vi "CreateFormatter.vi"(4 "Validate":bool=TRUE, 5 "DateFormat":string, 6 "Style":string, 7 "Format":string, 8 "error in (no error)":errorcluster, 10 "Name":string, 11 "Logger in":refnum<class "Logger.lvclass">) -> (0 "error out":errorcluster, 2 "Formatter":refnum<class "Formatter.lvclass">, 3 "Logger out":refnum<class "Logger.lvclass">)   [LabVIEW 2022 SP3, in "Logger.lvlib" / "Logger.lvclass"]
uses:
  Logger.lvclass
  C:/Users/jakub/repos/gh/sw4sys/lv-logger/PythonWrapper/Source/PythonSession/PythonSession.lvclass
  C:/Users/jakub/repos/gh/sw4sys/lv-logger/PythonWrapper/Source/PythonWrapper/PythonWrapper.lvclass
  C:/Users/jakub/repos/gh/sw4sys/lv-logger/Logger/Source/LoggingWrapper/LoggingWrapper.lvclass
  Formatter/Formatter.lvclass
  PythonWrapper/Source/PythonSession/PythonSession.lvclass/PythonSession.ctl
  PythonWrapper/Source/PythonWrapper/PythonWrapper.lvclass/PythonWrapper.ctl
  LoggingWrapper/LoggingWrapper.lvclass/LoggingWrapper.ctl
  Formatter/Formatter.lvclass/Formatter.ctl
  Formatter/Write Name.vi
  PythonWrapper/Source/PythonSession/Read PythonSession.vi
  PythonWrapper/Source/PythonWrapper/Read ModulePath.vi
  PythonWrapper/Source/PythonSession/SessionBank.vi
  Logger.lvclass/Logger.ctl
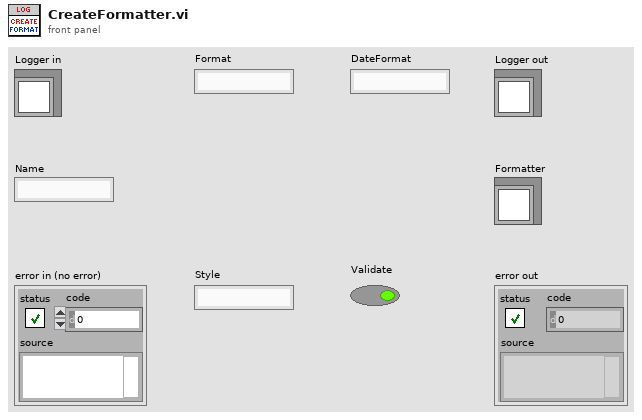
[diagram p1: front panel]
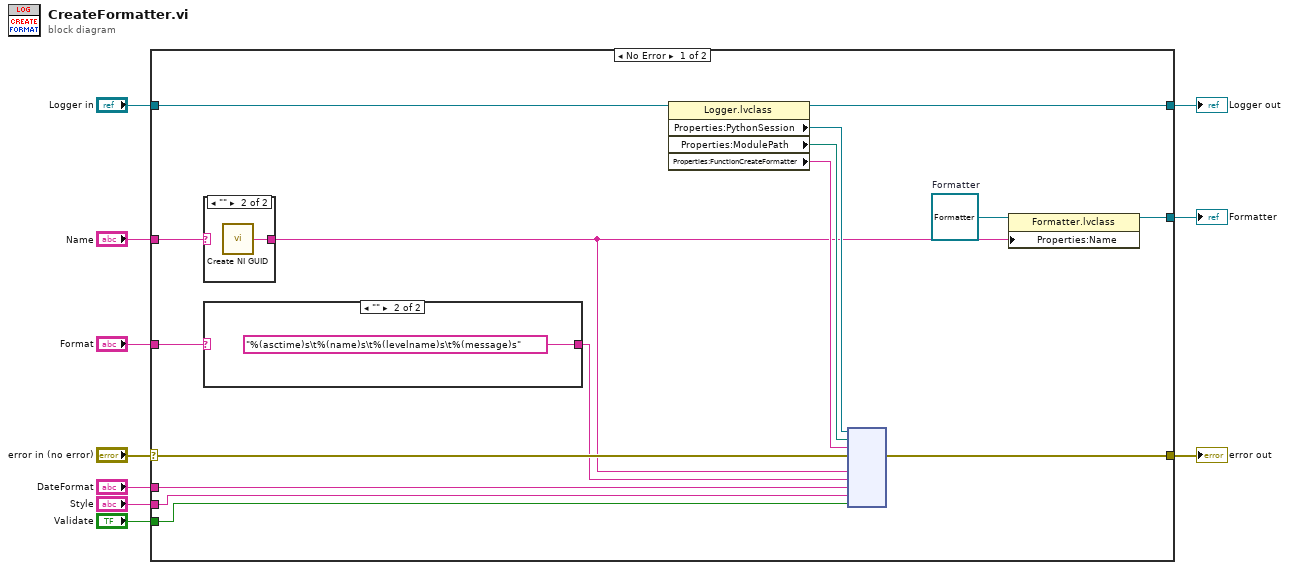
[diagram p0: block diagram]
diagram:
  n1 = case shown="No Error" "error in (no error)" {
    selector: "error in (no error)" -> [w20 w32]
    tunnel: [w19 w32] -> w6
    tunnel: [w17 w31] -> w8
    tunnel: "Logger in" -> [w22 w31]
    tunnel: "Format" -> [w21 _]
    tunnel: "DateFormat" -> [w13 _]
    tunnel: "Style" -> [w14 _]
    tunnel: "Validate" -> [w15 _]
    tunnel: [w16 _] -> w7
    tunnel: "Name" -> [w18 _]
    frame No Error {
      w23 = refnum<class "Formatter.lvclass"> refnum  # Formatter
      n2 = case shown="\"\"" w18 {
        selector: w18 -> [w29 _]
        tunnel: [w29 w30] -> w11
        frame Default {
        }
        frame "" {
          n3 = call <vilib>:"Create NI GUID.vi"() -> ("NI GUID"=w30:string)
        }
      }
      n4 = case shown="\"\"" w21 {
        selector: w21 -> [w27 _]
        tunnel: [w27 "%(asctime)s\t%(name)s\t%(levelname)s\t%(message)s"] -> w12
        frame Default {
        }
        frame "" {
        }
      }
      n5 = property class="Logger.lvclass"(reference=w22) -> (reference out=w17:refnum<class "Logger.lvclass">, "Properties:PythonSession"=w24:refnum<k35>, "Properties:ModulePath"=w26:path, "Properties:FunctionCreateFormatter"=w25:string)  [unwired: 1 in, 1 out]
      n6 = node(w24, w26, w25, w20, w11, w12, w13, w14, w15) -> (w19:errorcluster)  [unwired: 7 in, 3 out]
      n7 = property class="Formatter.lvclass"(reference=w23, "Properties:Name"=w11) -> (reference out=w16:refnum<class "Formatter.lvclass">)  [unwired: 1 in, 1 out]
    }
    frame Error {
    }
  }
  "error out" <- w6
  "Logger out" <- w8
  "Formatter" <- w7
